vi "myRIO_BRig_RT_comm_webdav_existFile.vi"(10 "input_fileName":string="dataTrial", 11 "input_hSession":T1) -> (1 "I_exist":bool)   [LabVIEW 2014]
uses:
  <vilib>/WebDAVClient/Advanced/SessionHandle.ctl
  <vilib>/WebDAVClient/NI_WebDAV.lvlib
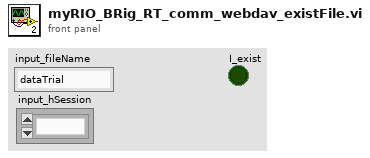
[diagram p1: front panel]
types:
  T1 = typedef "NI_WebDAV.lvlib/SessionHandle.ctl" = refnum<k1>
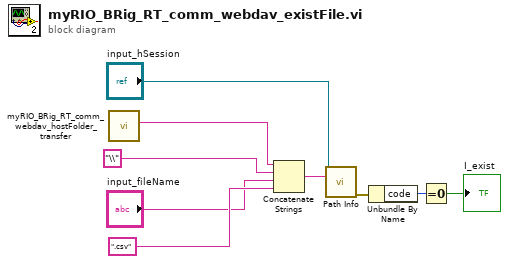
[diagram p0: block diagram]
diagram:
  n1 = call "myRIO_BRig_RT_comm_webdav_hostFolder_transfer.vi"() -> ("output_HostFolder"=w9:string)  [unwired: 11 in]
  n2 = Concatenate Strings(w9, "\\" ("string"), "input_fileName", ".csv" ("string")) -> (w5:string)
  n3 = call <vilib>:"Path Info.vi"("session handle"="input_hSession", "relative uri"=w5) -> ("error out"=w4:errorcluster)  [unwired: 10 in, 3 out]
  n4 = Unbundle By Name(w4) -> ("code"=w3:i32)
  n5 = Equal To 0?(x=w3) -> (x = 0?=→"I_exist":bool)
